vi "Read Name.vi"(8 "error in (no error)":errorcluster, 11 "Arduino Detector in":refnum<class "Arduino Detector.lvclass">) -> (0 "error out":errorcluster, 2 "Name":string, 3 "Arduino Detector out":refnum<class "Arduino Detector.lvclass">)   [LabVIEW 2019, in "Arduino Detector.lvclass"]
uses:
  Arduino Detector.lvclass
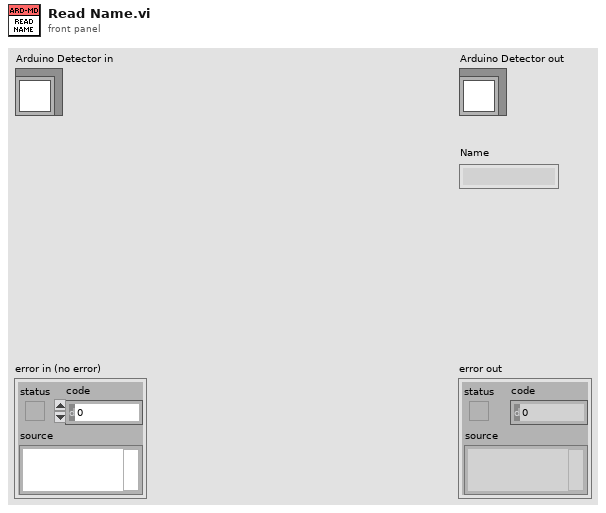
[diagram p1: front panel]
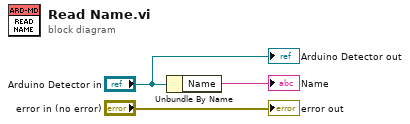
[diagram p0: block diagram]
diagram:
  n1 = Unbundle By Name("Arduino Detector in") -> ("Name"=→"Name":string)
  "error out" <- "error in (no error)"
  "Arduino Detector out" <- "Arduino Detector in"
